vi "ni579x Compare Versions.vi"(0 "Host Current Version":u32, 5 "Host Oldest Compatible Version":u32, 7 "FPGA Current Version":u32, 9 "FPGA Oldest Compatible Version":u32, 11 "Error In":errorcluster) -> (15 "Error Out":errorcluster)   [LabVIEW 2015, in "ni579x Config v2 Host.lvlib"]
uses:
  <instrlib>/ni579x/Config/v2/Host/ni579x Config v2 Host.lvlib
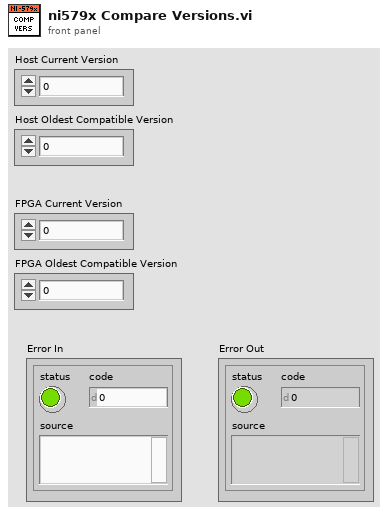
[diagram p1: front panel]
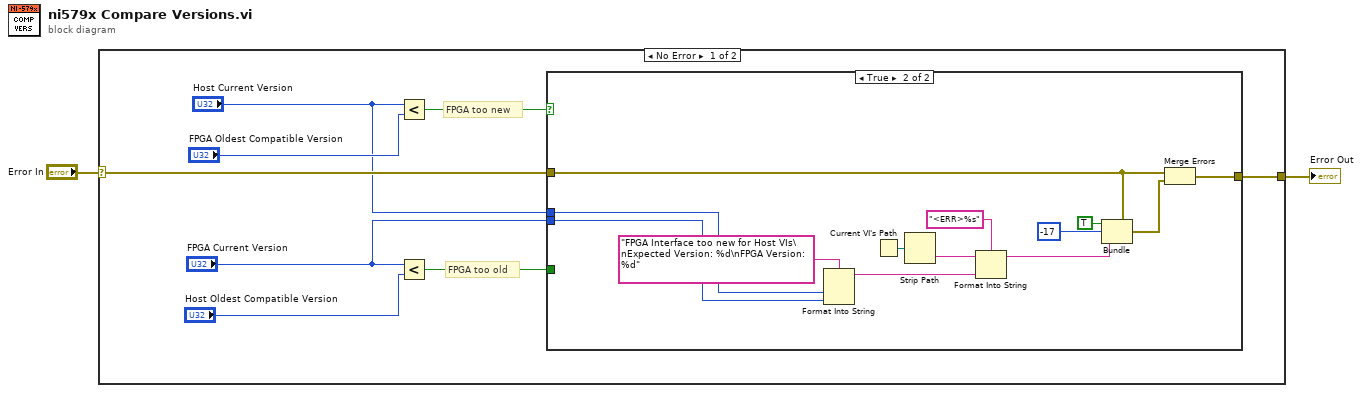
[diagram p0: block diagram]
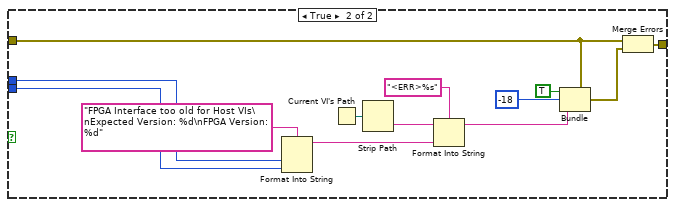
[diagram p3: hidden frame]
diagram:
  n1 = case shown="No Error" "Error In" {
    selector: "Error In" -> [w6 w43]
    tunnel: [w3 w43] -> w1
    frame No Error {
      # "FPGA too old"
      # "FPGA too new"
      n2 = Less?(x="Host Current Version", y="FPGA Oldest Compatible Version") -> (x < y?=w8:bool)
      n3 = Less?(x="FPGA Current Version", y="Host Oldest Compatible Version") -> (x < y?=w7:bool)
      n4 = case shown="True" w8 {
        tunnel: w7 -> [w15 _]
        tunnel: w6 -> [w14 w33]
        tunnel: "Host Current Version" -> [w12 w32]
        tunnel: "FPGA Current Version" -> [w11 w31]
        tunnel: [w13 w30] -> w3
        frame False {
          n5 = case shown="False" w15 {
            tunnel: w14 -> [w16 w20]
            tunnel: [w16 w19] -> w13
            tunnel: w12 -> [_ w18]
            tunnel: w11 -> [_ w17]
            frame False {
            }
            frame True {
              n6 = Format Into String(format string="FPGA Interface too old for Host VIs\nExpected Version: %d\nFPGA Version: %d" ("error message (\"\")"), w18, w17) -> (resulting string=w29:string)  [unwired: 2 in, 1 out]
              n7 = Current VI's Path() -> (path=w23:path)
              n8 = Strip Path(path=w23) -> (name=w24:string)  [unwired: 1 out]
              n9 = Format Into String(format string="<ERR>%s", initial string=w24, w29) -> (resulting string=w25:string)  [unwired: 1 in, 1 out]
              n10 = Bundle(cluster=w20, "status"=TRUE, "code"=-18, "source"=w25) -> (w26:errorcluster)
              n11 = Merge Errors(w20, w26) -> (w19:errorcluster)
            }
          }
        }
        frame True {
          n12 = Format Into String(format string="FPGA Interface too new for Host VIs\nExpected Version: %d\nFPGA Version: %d" ("error message (\"\")"), w32, w31) -> (resulting string=w42:string)  [unwired: 2 in, 1 out]
          n13 = Current VI's Path() -> (path=w36:path)
          n14 = Strip Path(path=w36) -> (name=w37:string)  [unwired: 1 out]
          n15 = Format Into String(format string="<ERR>%s", initial string=w37, w42) -> (resulting string=w38:string)  [unwired: 1 in, 1 out]
          n16 = Bundle(cluster=w33, "status"=TRUE, "code"=-17, "source"=w38) -> (w39:errorcluster)
          n17 = Merge Errors(w33, w39) -> (w30:errorcluster)
        }
      }
    }
    frame Error {
    }
  }
  "Error Out" <- w1
